vi "Release Queues.vi"(8 "error in (no error) in":errorcluster, 11 "Queues":T1) -> (0 "error out":errorcluster)   [LabVIEW 2017]
uses:
  Controls/Queues.ctl
  Controls/Frame Grabber State.ctl
  Controls/Optitrack State.ctl
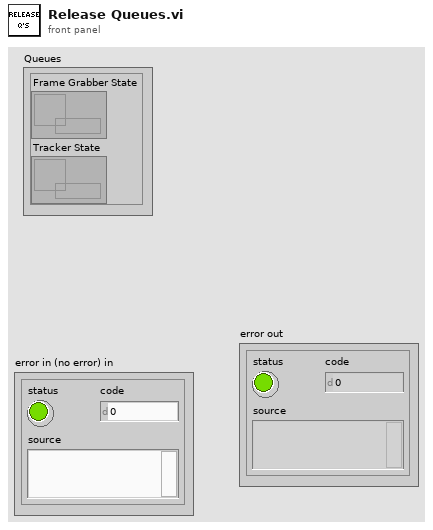
[diagram p1: front panel]
types:
  T1 = typedef "Queues.ctl" = cluster{"Frame Grabber State":refnum<queue>, "Tracker State":refnum<queue>}
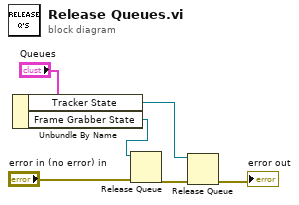
[diagram p0: block diagram]
diagram:
  n1 = Unbundle By Name("Queues") -> ("Tracker State"=w3:refnum<queue>, "Frame Grabber State"=w4:refnum<queue>)
  n2 = Release Queue(queue=w4, error in (no error)="error in (no error) in") -> (error out=w2:errorcluster)  [unwired: 1 in, 2 out]
  n3 = Release Queue(queue=w3, error in (no error)=w2) -> (error out=→"error out":errorcluster)  [unwired: 1 in, 2 out]
